vi "LVClasse_SurfaceFloatWithPupil Set Data.vi"(0 "SurfaceFloatWithPupil in":refnum<class "SurfaceFloatWithPupil.lvclass">, 5 "data":sgl[][](array[numeric]), 7 "Pupil":refnum<class "Pupil.lvclass">, 11 "error in (no error)":errorcluster) -> (4 "SurfaceFloatWithPupil out":refnum<class "SurfaceFloatWithPupil.lvclass">, 15 "error out":errorcluster)   [LabVIEW 2020, in "SurfaceFloatWithPupil.lvclass"]
doc: "Phase values buffer and cPupil setter.\n\n--------------------------------------------------------------------------------\n\n<B>PhaseIn</B> : Phase object.\n<B>PhaseOut</B> : Phase object.\n<B>data</B> : Phase values buffer.\n<B>Pupil</B> : cPupil object.\n<B>ErrorIn</B> : Error\n<B>ErrorOut</B> : Error\n\n--------------------------------------------------------------------------------"
uses:
  SurfaceFloatWithPupil.lvclass
  Pupil.lvclass
  SurfaceFloatWithPupil.lvclass/SurfaceFloatWithPupil.ctl
  LVClass_Pupil Read Pupil.vi
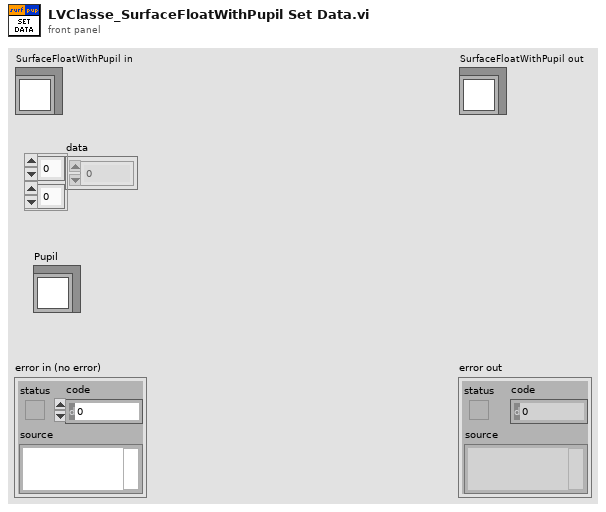
[diagram p1: front panel]
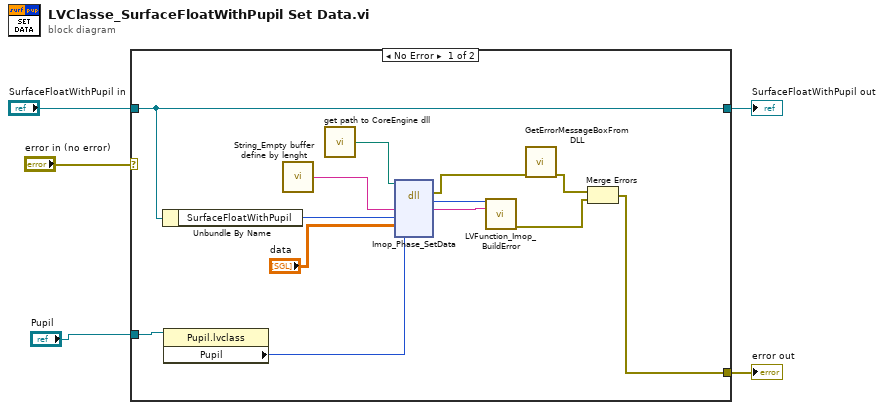
[diagram p0: block diagram]
diagram:
  n1 = case shown="No Error" "error in (no error)" {
    selector: "error in (no error)" -> [_ w20]
    tunnel: [w6 w20] -> w5
    tunnel: [w13 w19] -> w4
    tunnel: "SurfaceFloatWithPupil in" -> [w13 w19]
    tunnel: "Pupil" -> [w11 _]
    frame No Error {
      n2 = Unbundle By Name(w13) -> ("SurfaceFloatWithPupil"=w12:i32)
      n3 = property class="Pupil.lvclass"(reference=w11) -> ("Pupil"=w10:i32)  [unwired: 1 in, 2 out]
      n4 = call "String_Empty buffer define by lenght.vi"() -> ("Empty buffer"=w16:string)  [unwired: 1 in]
      n5 = call "get path to CoreEngine dll.vi"() -> ("path to c_interface_vc100.dll"=w15:path)  [unwired: 12 in, 3 out]
      n6 = dll-call lib="D:/2_trunk/Soft_haso/ImOpCoreEngine4_LV2011/DLLs/ImopEngine4_vc100.dll" fn="Imop_Phase_SetData"(path in=w15, "message"=w16, "phase"=w12, "data"="data", "pupil"=w10) -> (error out=w14:errorcluster, "return type"=w18:i32, "message"=w17:string)  [unwired: 5 in, 1 out]
      n7 = call "LVFunction_Imop_BuildError.vi"("code"=w18, "String to Prepend to source (\"\")"=w17) -> ("error out"=w7:errorcluster)  [unwired: 13 in]
      n8 = call "GetErrorMessageBoxFromDLL.vi"("error IN"=w14) -> ("error OUT"=w8:errorcluster)  [unwired: 10 in]
      n9 = Merge Errors(w8, w7) -> (w6:errorcluster)
    }
    frame Error {
    }
  }
  "error out" <- w5
  "SurfaceFloatWithPupil out" <- w4
